vi "Handle.vi"(8 "error in (no error)":errorcluster, 11 "TelFocus in":refnum<class "TelFocus.lvclass">) -> (0 "error out":errorcluster, 3 "TelFocus out":refnum<class "TelFocus.lvclass">)   [LabVIEW 2018, in "TelFocus.lvclass"]
uses:
  TelFocus.lvclass
  TelFocus.lvclass/TelFocus.ctl
  Device/Device.lvclass/Device.ctl
  SecMirror/SecMirror.lvclass
  C:/Users/orlando/Documents/Orlando/SPARC4/Sparc4GUI/Versao ZeroMQ REQ-REP/SPARC4_GUI -v1.0.6 - set suffix automatico para os ACS/Device/Device.lvclass
  Server/Server.lvclass
  Comm/Stream/Stream.lvclass
  Device/Device.lvclass
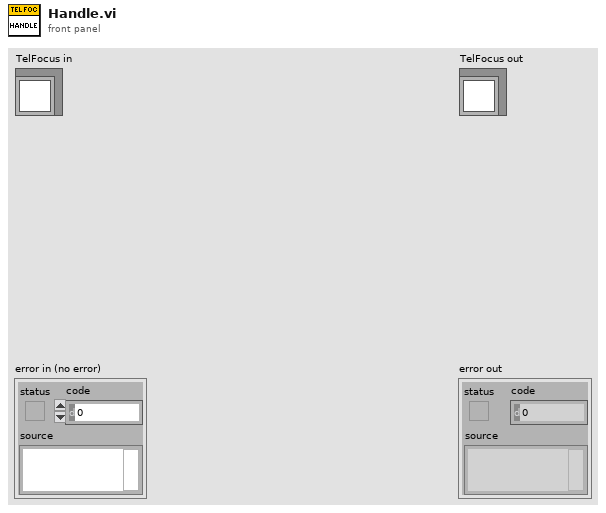
[diagram p1: front panel]
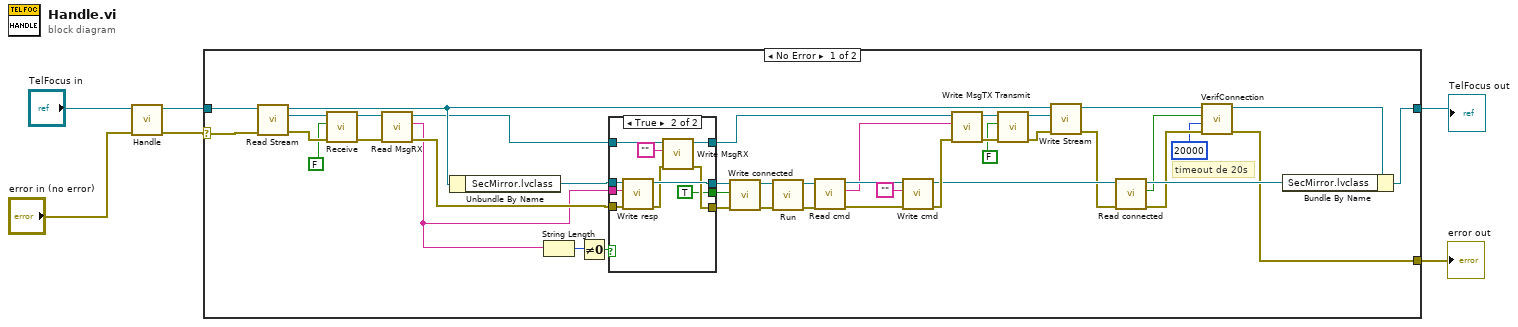
[diagram p0: block diagram]
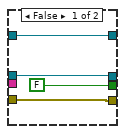
[diagram p2: hidden frame]
diagram:
  n1 = call-parent "Handle.vi"("error in (no error)"="error in (no error)", "Server in"="TelFocus in") -> ("error out"=w3:errorcluster, "Server out"=w4:refnum<class "TelFocus.lvclass">)  [unwired: 8 in]
  n2 = case shown="No Error" w3 {
    selector: w3 -> [w46 w64]
    tunnel: [w20 w64] -> w1
    tunnel: [w45 w63] -> w2
    tunnel: w4 -> [w37 w63]
    frame No Error {
      # "timeout de 20s"
      n3 = call-dynamic "Read Stream.vi"("error in (no error)"=w46, "Server in"=w37) -> ("error out"=w47:errorcluster, "Stream.lvclass"=w48:refnum<class "Stream.lvclass">, "Server out"=w39:refnum<class "TelFocus.lvclass">)  [unwired: 7 in]
      n4 = call-dynamic "Receive.vi"("error in (no error)"=w47, "log?"=FALSE, "Stream in"=w48) -> ("error out"=w44:errorcluster, "Stream out"=w43:refnum<class "Stream.lvclass">)  [unwired: 7 in]
      n5 = call-dynamic "Read MsgRX.vi"("error in (no error)"=w44, "Comm in"=w43) -> ("error out"=w17:errorcluster, "MsgRX"=w16:string, "Comm out"=w15:refnum<class "Stream.lvclass">)  [unwired: 7 in]
      n6 = Unbundle By Name(w39) -> ("SecMirror.lvclass"=w18:refnum<class "SecMirror.lvclass">)
      n7 = String Length(string=w16) -> (length=w31:i32)
      n8 = Not Equal To 0?(x=w31) -> (x != 0?=w30:bool)
      n9 = case shown="True" w30 {
        tunnel: [w51 w55] -> w11
        tunnel: [w52 w61] -> w12
        tunnel: w17 -> [w51 w60]
        tunnel: w18 -> [w52 w62]
        tunnel: w16 -> [_ w59]
        tunnel: w15 -> [w50 w58]
        tunnel: [w50 w57] -> w14
        tunnel: [FALSE TRUE] -> w13
        frame False {
        }
        frame True {
          n10 = call-dynamic "Write resp.vi"("error in (no error)"=w60, "resp"=w59, "Device in"=w62) -> ("error out"=w56:errorcluster, "Device out"=w61:refnum<class "SecMirror.lvclass">)  [unwired: 7 in]
          n11 = call-dynamic "Write MsgRX.vi"("error in (no error)"=w56, "MsgRX"="", "Comm in"=w58) -> ("error out"=w55:errorcluster, "Comm out"=w57:refnum<class "Stream.lvclass">)  [unwired: 7 in]
        }
      }
      n12 = call "Write connected.vi"("error in (no error)"=w11, "connected"=w13, "Device in"=w12) -> ("error out"=w9:errorcluster, "Device out"=w10:refnum<class "SecMirror.lvclass">)  [unwired: 7 in]
      n13 = call-dynamic "Run.vi"("error in (no error)"=w9, "SecMirror in"=w10) -> ("error out"=w28:errorcluster, "SecMirror out"=w29:refnum<class "SecMirror.lvclass">)  [unwired: 8 in]
      n14 = call-dynamic "Read cmd.vi"("error in (no error)"=w28, "Device in"=w29) -> ("error out"=w35:errorcluster, "cmd"=w33:string, "Device out"=w36:refnum<class "SecMirror.lvclass">)  [unwired: 7 in]
      n15 = call-dynamic "Write cmd.vi"("error in (no error)"=w35, "cmd"="", "Device in"=w36) -> ("error out"=w42:errorcluster, "Device out"=w27:refnum<class "SecMirror.lvclass">)  [unwired: 7 in]
      n16 = call-dynamic "Write MsgTX.vi"("error in (no error)"=w42, "MsgTX"=w33, "Comm in"=w14) -> ("error out"=w40:errorcluster, "Comm out"=w41:refnum<class "Stream.lvclass">)  [unwired: 7 in]
      n17 = call-dynamic "Transmit.vi"("error in (no error)"=w40, "log?"=FALSE, "Stream in"=w41) -> ("error out"=w38:errorcluster, "Stream out"=w32:refnum<class "Stream.lvclass">)  [unwired: 7 in]
      n18 = call-dynamic "Write Stream.vi"("error in (no error)"=w38, "Stream.lvclass"=w32, "Server in"=w39) -> ("error out"=w26:errorcluster, "Server out"=w25:refnum<class "TelFocus.lvclass">)  [unwired: 7 in]
      n19 = call "Read connected.vi"("error in (no error)"=w26, "Device in"=w27) -> ("error out"=w21:errorcluster, "connected"=w23:bool, "Device out"=w24:refnum<class "SecMirror.lvclass">)  [unwired: 7 in]
      n20 = call-dynamic "VerifConnection.vi"("error in (no error)"=w21, "timeout in ms (1000)"=u32 20000 ("period (ms)"), "device connected in"=w23, "Server in"=w25) -> ("error out"=w20:errorcluster, "Server out"=w22:refnum<class "TelFocus.lvclass">)  [unwired: 6 in]
      n21 = Bundle By Name(cluster=w22, "SecMirror.lvclass"=w24) -> (w45:refnum<class "TelFocus.lvclass">)
    }
    frame Error {
    }
  }
  "error out" <- w1
  "TelFocus out" <- w2
